vi "Fine Thresholding.vi"(4 "Fine Threshold Parameters":T7={"Current"=[20, 20, 20, 20, 20], "Pulse Duration"=[500, 500, 500, 500], "Train Length"=[200, 200, 200, 200, 200, 114, 214, 314, 414, 514]} {"Train Length" min=20 max=500 step=5}, 5 "Stimulator":T1={"Stim Open Data"={"Name"="", "Mode"=enum."LIVE", "Visa Timeout"=0}, "Stim Init Data"={"Frequency"=0.0, "N Factor"=0, "D/T Int"=0.0, "Active Channels"=[], "LF Channels"=[]}, "Stim Update Data"={"Pulse Mode"=[enum."Single"], "Current"=[], "Pulse Dur"=[]}, "Stim Status"={"Open"=FALSE, "On"=FALSE}}) -> (1 "Fine Threshold Parameters":T7={"Current"=[20, 20, 20, 20, 20], "Pulse Duration"=[500, 500, 500, 500], "Train Length"=[200, 200, 200, 200, 200, 114, 214, 314, 414, 514]} {"Train Length" min=20 max=500 step=5}, 2 "Stimulator":T1={"Stim Open Data"={"Name"="", "Mode"=enum."LIVE", "Visa Timeout"=0}, "Stim Init Data"={"Frequency"=0.0, "N Factor"=0, "D/T Int"=0.0, "Active Channels"=[], "LF Channels"=[]}, "Stim Update Data"={"Pulse Mode"=[enum."Single"], "Current"=[], "Pulse Dur"=[]}, "Stim Status"={"Open"=FALSE, "On"=FALSE}})   [LabVIEW 2019]
uses:
  Data Type Defs/Stimulator.ctl
  Data Type Defs/Stim Open Data.ctl
  Data Type Defs/Stim Init Data.ctl
  Data Type Defs/Stim Update Data.ctl
  Data Type Defs/Pulse Mode (array).ctl
  Data Type Defs/Stim Status.ctl
  Controls/Type Defs/Fine Tuning Threshold Params.ctl
  Controls/Stim Current Array.ctl
  Controls/Pulse Duration Array.ctl
  Controls/Train Length Array.ctl
  Controls/Type Defs/Single Channel Params.ctl
panel:
  out "Stim Train Log String":string
  in  "Train Length":u16[](array[numeric]) caption="Train Length (ms)" max=1000 step=5
  in  "Current":u16[](array[numeric]) caption="Current (mA)" max=126 step=2
  in  "PW":u16[](array[numeric]) caption="PW (us)" min=20 max=500 step=5
  in  "Channel":bool[](array[boolean])=[FALSE, FALSE, FALSE, FALSE, FALSE]
  in  "Done":bool
  # "Gluteals"
  # "Hamstrings"
  # "Quads"
  # "TA/Dorsi"
  # "TS/Plantar"
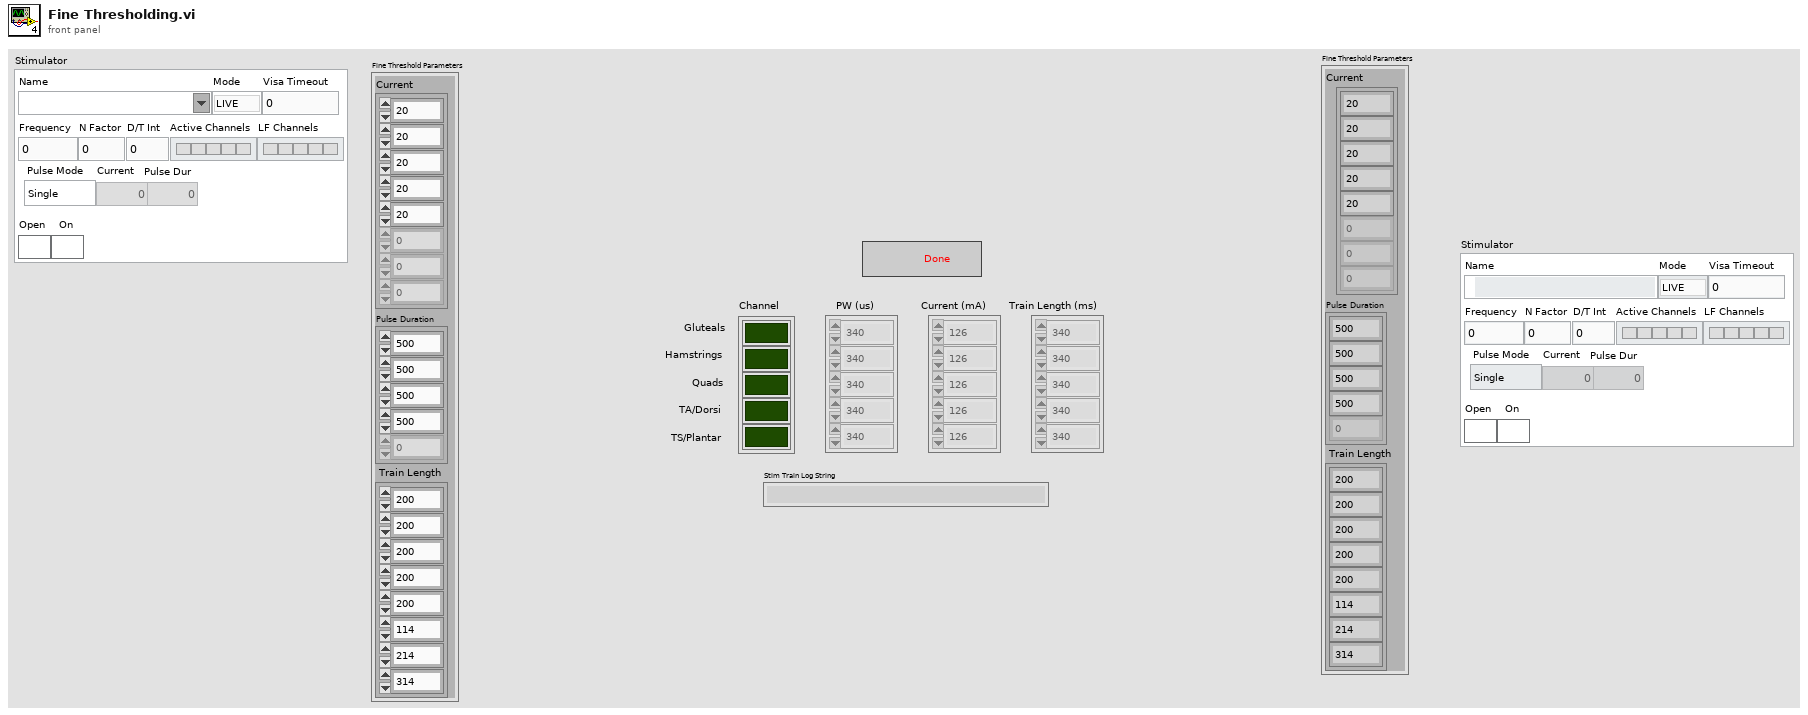
[diagram p1: front panel]
types:
  T1 = typedef "Stimulator.ctl" = cluster{"Stim Open Data":T2, "Stim Init Data":T3, "Stim Update Data":T4, "Stim Status":T6}
  T2 = typedef "Stim Open Data.ctl" = cluster{"Name":refnum<visa-resource-name>, "Mode":enum16{"LIVE", "SIM"}, "Visa Timeout":u32}
  T3 = typedef "Stim Init Data.ctl" = cluster{"Frequency":dbl, "N Factor":u8, "D/T Int":dbl, "Active Channels":bool[], "LF Channels":bool[]}
  T4 = typedef "Stim Update Data.ctl" = cluster{"Pulse Mode":T5, "Current":u32[], "Pulse Dur":u32[]}
  T5 = typedef "Pulse Mode (array).ctl" = enum16{"Single", "Doublet", "Triplet"}[]
  T6 = typedef "Stim Status.ctl" = cluster{"Open":bool, "On":bool}
  T7 = typedef "Fine Tuning Threshold Params.ctl" = cluster{"Current":T8, "Pulse Duration":T9, "Train Length":T10}
  T8 = typedef "Stim Current Array.ctl" = u8[]
  T9 = typedef "Pulse Duration Array.ctl" = u32[]
  T10 = typedef "Train Length Array.ctl" = i64[]
  T11 = typedef "Single Channel Params.ctl" = cluster{"Channel":i32, "Current":u8, "Pulse duration":u16, "Train Length":i64}
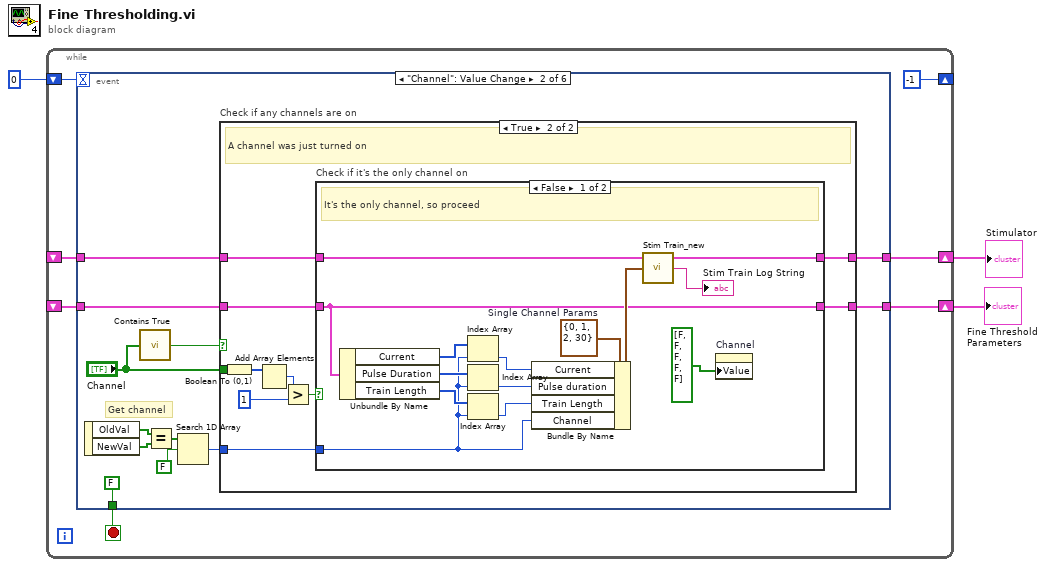
[diagram p0: block diagram]
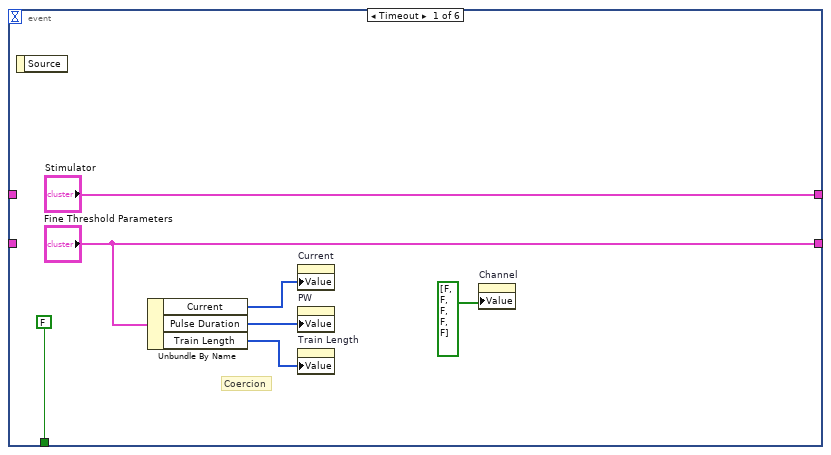
[diagram p2: hidden frame]
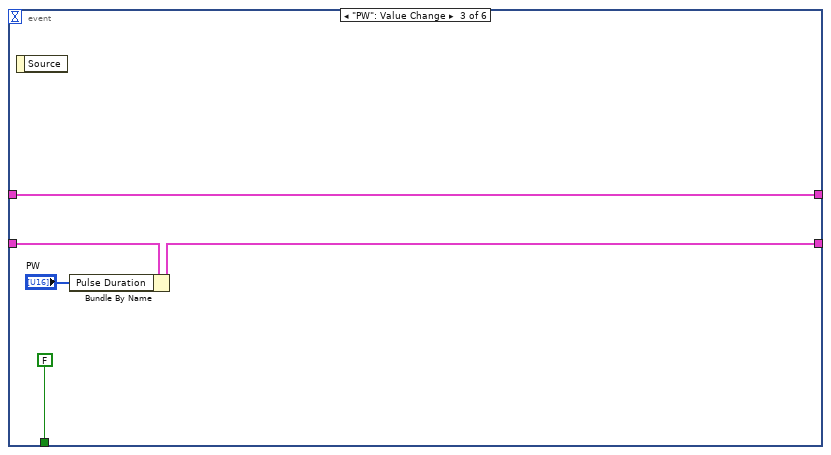
[diagram p5: hidden frame]
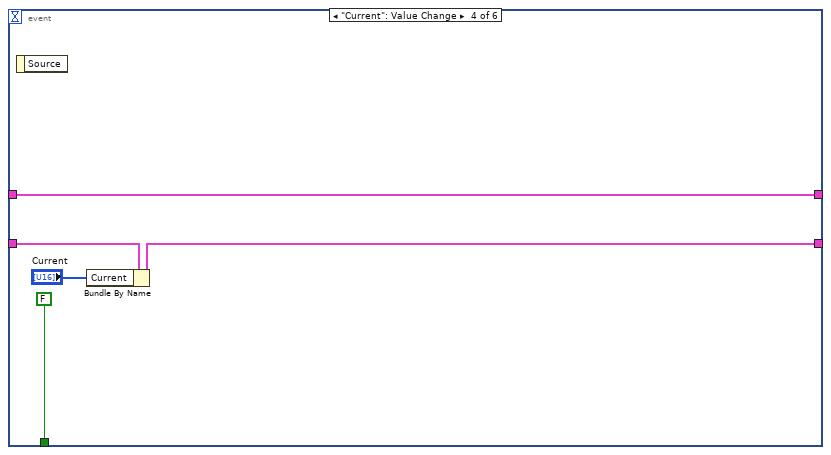
[diagram p6: hidden frame]
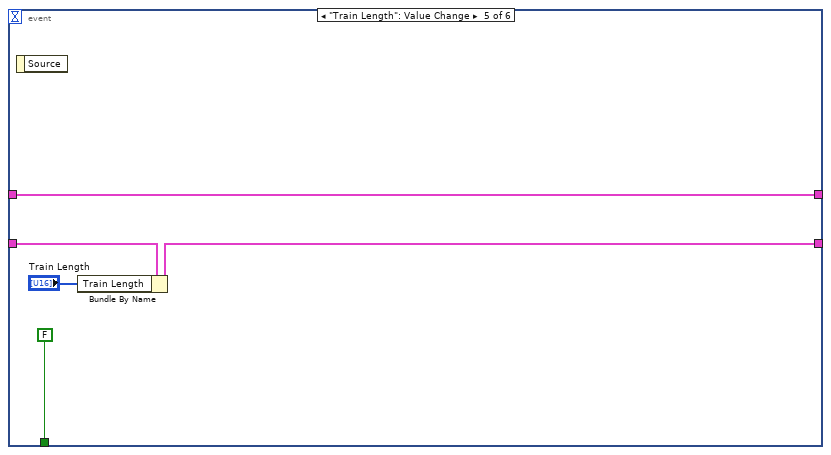
[diagram p7: hidden frame]
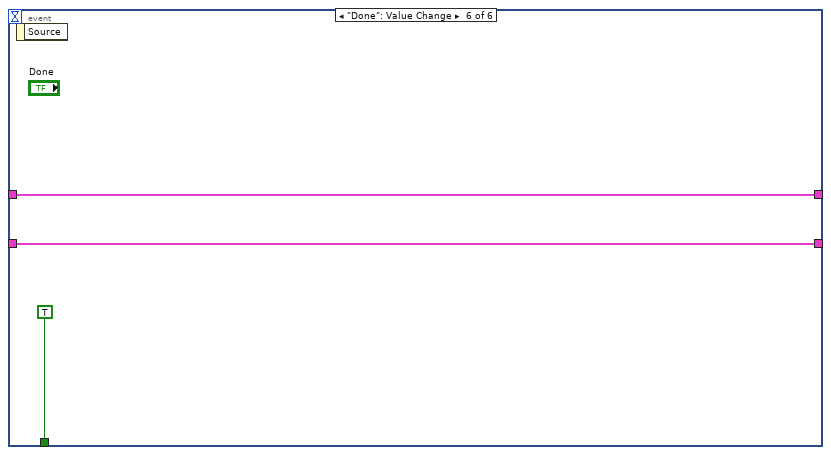
[diagram p8: hidden frame]
diagram:
  n1 = while "Stim Loop" {
    shift-right: [-1] -> _
    shift-left: 0 -> [w9]
    shift-right: [w7] -> w2
    shift-left: _ -> [w6]
    shift-right: [w5] -> w1
    shift-left: _ -> [w4]
    stop <- w10 stop-if-true
    n2 = event shown="[1] \"Channel\": Value Change" {
      selector: _ -> [_ _ _ _ _ _]
      dyn-events: _ -> [_ _ _ _ _ _]
      timeout: w9 -> [_ _ _ _ _ _]
      tunnel: [FALSE FALSE FALSE FALSE FALSE TRUE] -> w10
      tunnel: ["Fine Threshold Parameters" w18 w61 w65 w70 w74] -> w7
      tunnel: w6 -> [_ w21 w62 w66 w71 w74]
      tunnel: ["Stimulator" w20 w59 w63 w68 w73] -> w5
      tunnel: w4 -> [_ w22 w59 w63 w68 w73]
      event Timeout {
        # "Coercion"
        n3 = event-data() -> ()  [unwired: 1 in, 1 out]
        n4 = Unbundle By Name("Fine Threshold Parameters") -> ("Current"=w16:T8, "Pulse Duration"=w13:T9, "Train Length"=w15:T10)
        n5 = property on="Current" class="Arr (strict)"("Value"=w16) -> ()  [unwired: 2 in, 2 out]
        n6 = property on="PW" class="Arr (strict)"("Value"=w13) -> ()  [unwired: 2 in, 2 out]
        n7 = property on="Train Length" class="Arr (strict)"("Value"=w15) -> ()  [unwired: 2 in, 2 out]
        n8 = property on="Channel" class="Arr (strict)"("Value"=bool[] [FALSE, FALSE, FALSE, FALSE, FALSE] ("Channel")) -> ()  [unwired: 2 in, 2 out]
      }
      event "Channel": Value Change {
        # "Get channel"
        n9 = event-data() -> ("OldVal"=w26:bool[], "NewVal"=w25:bool[])  [unwired: 1 in]
        n10 = call "Contains True.vi"("R Channel BL"="Channel") -> ("Boolean"=w28:bool)
        n11 = Equal?(x=w26, y=w25) -> (x = y?=w24:bool[])
        n12 = Search 1D Array(1D array=w24, element=FALSE) -> (index of element=w23:i32)  [unwired: 1 in]
        n13 = case "Check if any channels are on" shown="True" w28 {
          tunnel: "Channel" -> [_ w37]
          tunnel: w23 -> [_ w36]
          tunnel: w22 -> [w31 w34]
          tunnel: w21 -> [w30 w35]
          tunnel: [w31 w33] -> w20
          tunnel: [w30 w32] -> w18
          frame False {
            # "I don't think this happens."
            # "A channel was just turned off"
          }
          frame True {
            # "A channel was just turned on"
            n14 = Boolean To (0,1)(Boolean=w37) -> (0, 1=w41:i16[])
            n15 = Add Array Elements(numeric array=w41) -> (sum=w40:i16)
            n16 = Greater?(x=w40, y=i16 1) -> (0:w38:bool)
            n17 = case "Check if it's the only channel on" shown="False" w38 {
              tunnel: w36 -> [w42 _]
              tunnel: w35 -> [w43 w56]
              tunnel: w34 -> [w54 w57]
              tunnel: [w45 w57] -> w33
              tunnel: [w43 w56] -> w32
              frame False {
                w50 = T11 {"Channel"=0, "Current"=1, "Pulse duration"=2, "Train Length"=30}  # Single Channel Params
                # "It's the only channel, so proceed"
                n18 = Unbundle By Name(w43) -> ("Current"=w53:T8, "Pulse Duration"=w51:T9, "Train Length"=w52:T10)
                n19 = Index Array(array=w53, index=w42) -> (element=w48:u8)
                n20 = Index Array(array=w51, index=w42) -> (element=w47:u32)
                n21 = Index Array(array=w52, index=w42) -> (element=w46:i64)
                n22 = Bundle By Name(cluster=w50, "Current"=w48, "Pulse duration"=w47, "Train Length"=w46, "Channel"=w42) -> (w49:T11)
                n23 = call "Stim Train_new.vi"("Single Channel Params"=w49, "Stimulator"=w54) -> ("Stim Train Log String"=→"Stim Train Log String":string, "Stimulator Out"=w45:T1)  [unwired: 2 in]
                n24 = property on="Channel" class="Arr (strict)"("Value"=bool[] [FALSE, FALSE, FALSE, FALSE, FALSE] ("Channel")) -> ()  [unwired: 2 in, 2 out]
              }
              frame True {
                # "There's already a channel on, so ignore the new one"
              }
            }
          }
        }
      }
      event "PW": Value Change {
        n25 = event-data() -> ()  [unwired: 1 in, 1 out]
        n26 = Bundle By Name(cluster=w62, "Pulse Duration"="PW") -> (w61:T7)
      }
      event "Current": Value Change {
        n27 = event-data() -> ()  [unwired: 1 in, 1 out]
        n28 = Bundle By Name(cluster=w66, "Current"="Current") -> (w65:T7)
      }
      event "Train Length": Value Change {
        n29 = event-data() -> ()  [unwired: 1 in, 1 out]
        n30 = Bundle By Name(cluster=w71, "Train Length"="Train Length") -> (w70:T7)
      }
      event "Done": Value Change {
        n31 = event-data() -> ()  [unwired: 1 in, 1 out]
      }
    }
  }
  "Fine Threshold Parameters" <- w2
  "Stimulator" <- w1
